vi "Circulate.vi"(6 "Robot":refnum<class "Robot.lvclass">, 8 "error in (no error)":errorcluster, 9 "Clockwise?":bool, 10 "Target":dbl[](array[numeric]), 11 "CirculateSkill in":refnum<class "CirculateSkill.lvclass">) -> (0 "error out":errorcluster, 1 "Robot out":refnum<class "Robot.lvclass">, 3 "CirculateSkill out":refnum<class "CirculateSkill.lvclass">)   [LabVIEW 2023, in "CirculateSkill.lvclass"]
uses:
  CirculateSkill.lvclass
  C:/Users/ebert/Documents/codes/SSL/repo/SSL_AI/GoToSkill_class/GoToSkill.lvclass
  Robot_class/Robot.lvclass
  C:/Users/ebert/Documents/codes/SSL/repo/SSL_AI/Object_class/Object.lvclass
  Object_class/Object.lvclass/Object.ctl
  <vilib>/Analysis/_algsub.llb/Real Vector Norm.vi
  Object_class/Read position(x,y).vi
  GoToSkill_class/GoToSkill.lvclass
  <vilib>/Analysis/NI_AALPro.lvlib
panel:
  in  "radial factor":dbl
  in  "tangent factor":dbl=0.2 format="%#_13g"
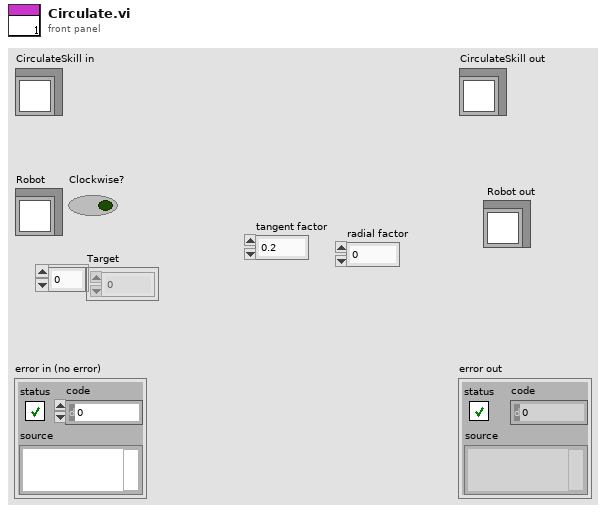
[diagram p1: front panel]
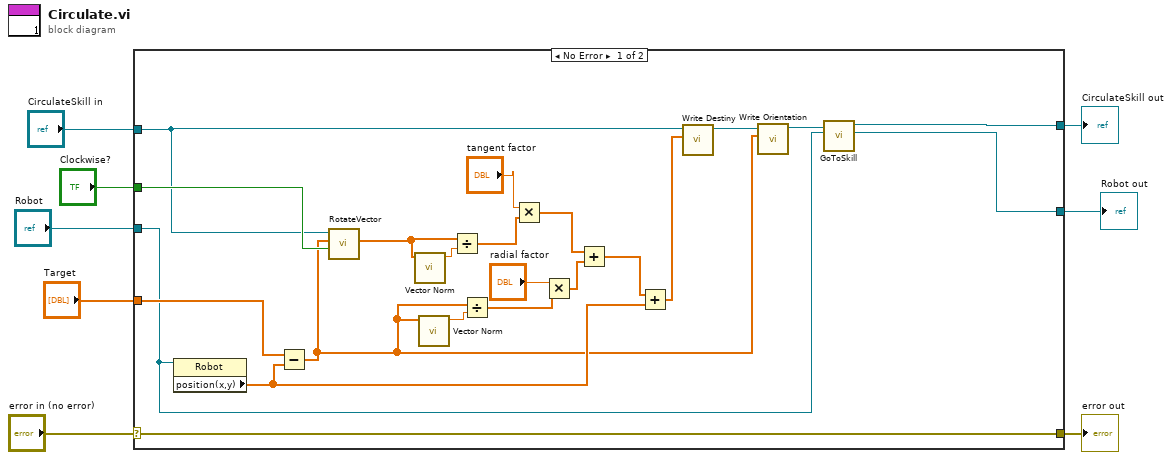
[diagram p0: block diagram]
diagram:
  n1 = case shown="No Error" "error in (no error)" {
    selector: "error in (no error)" -> [w30 w33]
    tunnel: [w30 w33] -> w7
    tunnel: [w28 w32] -> w5
    tunnel: "CirculateSkill in" -> [w21 w32]
    tunnel: "Robot" -> [w9 w31]
    tunnel: [w19 w31] -> w1
    tunnel: "Target" -> [w27 _]
    tunnel: "Clockwise?" -> [w26 _]
    frame No Error {
      n2 = property class="Robot"(reference=w9) -> ("position(x,y)"=w22:dbl[])  [unwired: 1 in, 2 out]
      n3 = Subtract(x=w27, y=w22) -> (x-y=w15:dbl[])
      n4 = call "RotateVector.vi"("Clockwise?"=w26, "Vector in"=w15, "CirculateSkill in"=w21) -> ("Vector out"=w25:dbl[])  [unwired: 6 in, 2 out]
      n5 = call-poly <vilib>:"Vector Norm.vi"("Input Vector"=w25) -> ("norm"=w24:dbl)  [unwired: 9 in, 1 out]
      n6 = call-poly <vilib>:"Vector Norm.vi"("Input Vector"=w15) -> ("norm"=w16:dbl)  [unwired: 9 in, 1 out]
      n7 = Divide(x=w25, y=w24) -> (x/y=w18:dbl[])
      n8 = Divide(x=w15, y=w16) -> (x/y=w14:dbl[])
      n9 = Multiply(x="tangent factor", y=w18) -> (x*y=w17:dbl[])
      n10 = Multiply(x="radial factor", y=w14) -> (x*y=w11:dbl[])
      n11 = Add(x=w17, y=w11) -> (x+y=w10:dbl[])
      n12 = Add(x=w10, y=w22) -> (x+y=w23:dbl[])
      n13 = call-dynamic "Write Destiny.vi"("Destiny"=w23, "GoToSkill in"=w21) -> ("GoToSkill out"=w29:refnum<class "CirculateSkill.lvclass">)  [unwired: 8 in, 1 out]
      n14 = call-dynamic "Write Orientation.vi"("Orientation"=w15, "GoToSkill in"=w29) -> ("GoToSkill out"=w20:refnum<class "CirculateSkill.lvclass">)  [unwired: 8 in, 1 out]
      n15 = call "GoToSkill.vi"("Robot"=w9, "GoToSkill in"=w20) -> ("Robot out"=w19:refnum<class "Robot.lvclass">, "GoToSkill out"=w28:refnum<class "CirculateSkill.lvclass">)  [unwired: 7 in, 1 out]
    }
    frame Error {
    }
  }
  "error out" <- w7
  "CirculateSkill out" <- w5
  "Robot out" <- w1
